vi "OFET.vi"() -> ()   [LabVIEW 2017]
uses:
  EnumEstados1.ctl
  <vilib>/Analysis/3filter.llb/Filter Passband Type.ctl
  <vilib>/Analysis/baseanly.llb/IIR Cascade Filter (DBL).vi
  <vilib>/Analysis/NI_AALBase.lvlib
  <vilib>/Utility/NIReport.llb/NI_report.lvclass
  <vilib>/addons/_office/NI_ReportGenerationToolkit.lvlib
  <vilib>/addons/_office/excel.llb/Excel Easy Table (str).vi
panel:
  in  "Tab Control":T1(tab)
  in  "Voltaje final:  2":dbl
  in  "Voltaje inicial:  2":dbl
  in  "Paso: 2":dbl
  in  "Voltaje final:":dbl
  in  "Voltaje inicial:":dbl
  in  "Paso:":dbl
  in  "Paso":dbl
  in  "Voltaje inicial:":dbl
  in  "Voltaje final:":dbl
  in  "Voltaje:":dbl
  in  "order":i32
  in  "Stop Button":bool
  in  "Save Button":bool
  in  "Guardar en:":path
  out "Voltage-Current Characterization:":cluster{dbl[], "Filtered X":dbl[]}(graph)
  in  "Ok":bool
  # "OFET"
  # "VGS"
  # "VDS"
  # "VGS"
  # "VDS"
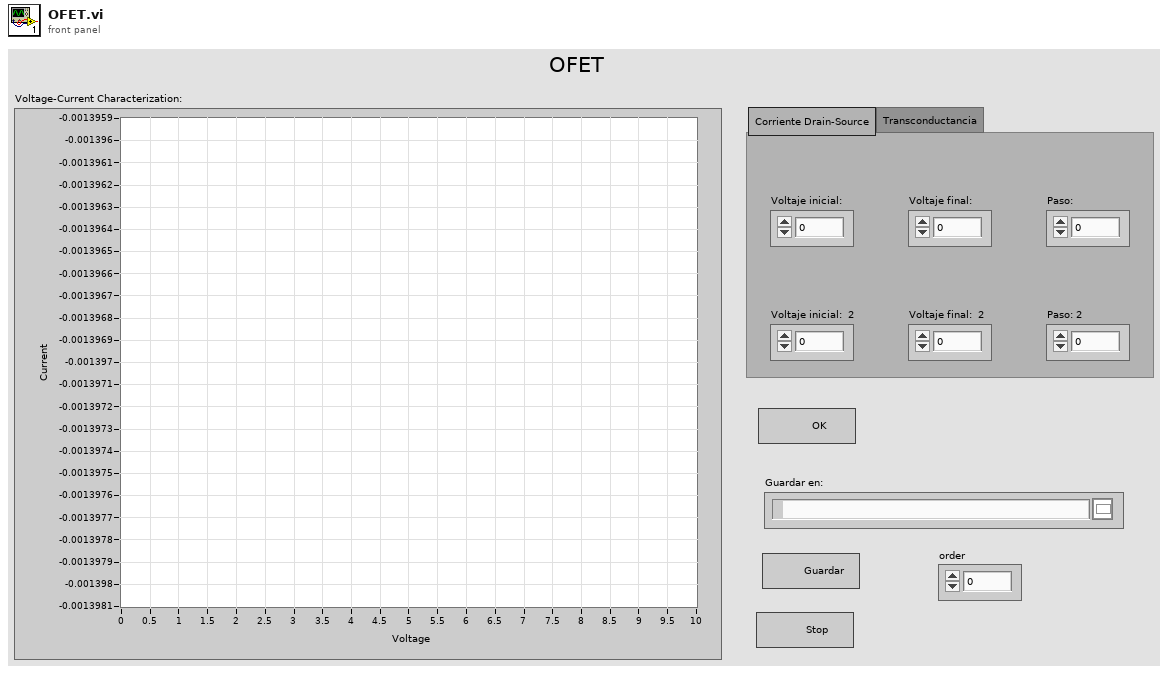
[diagram p1: front panel]
types:
  T1 = enum32{"Corriente Drain-Source", "Transconductancia"}
  T2 = typedef "EnumEstados1.ctl" = enum16{"Inicio", "LecturaDatos", "Cierre"}
  T3 = typedef "NI_AALBase.lvlib/Filter Passband Type.ctl" = enum32{"Lowpass", "Highpass", "Bandpass", "Bandstop"}
  T4 = enum16{"Standard Report", "HTML", "Word", "Excel"}
  T5 = enum16{"maximized", "minimized", "normal", "no change"}
  T6 = enum16{"open", "open or create", "create or replace", "create", "open (read-only)"}
  T7 = cluster{"task out":refnum<k21>, "error out":errorcluster}
  T8 = cluster{"filter structure":enum32{"IIR 2nd Order", "IIR 4th Order"}, "Reverse Coefficients":dbl[], "Forward Coefficients":dbl[]}
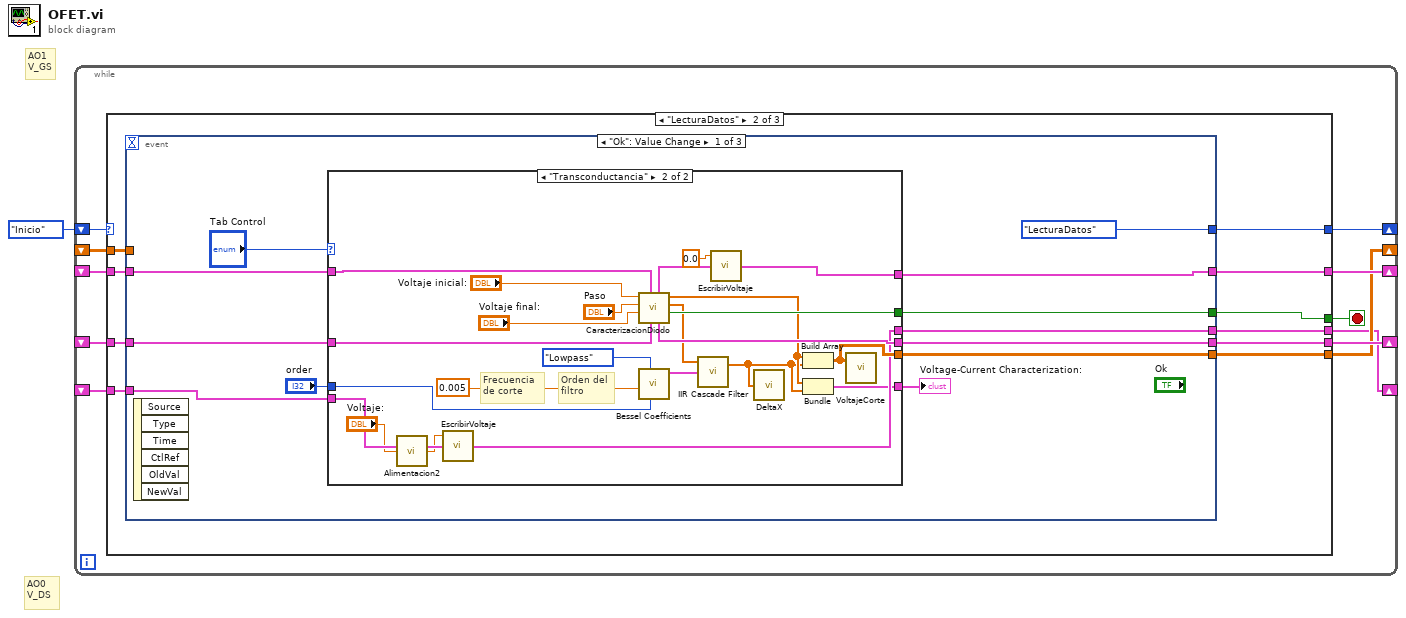
[diagram p0: block diagram]
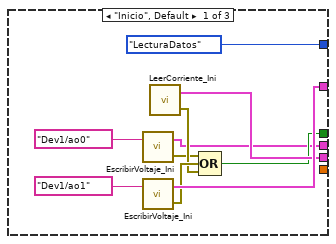
[diagram p2: hidden frame]
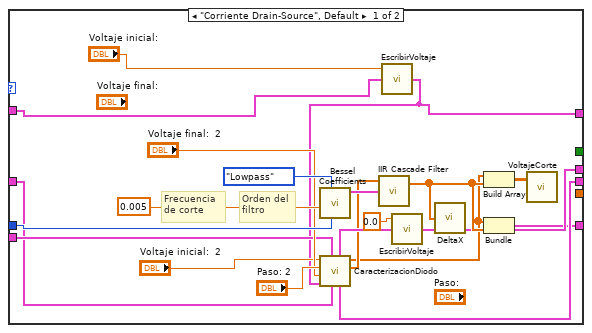
[diagram p3: hidden frame]
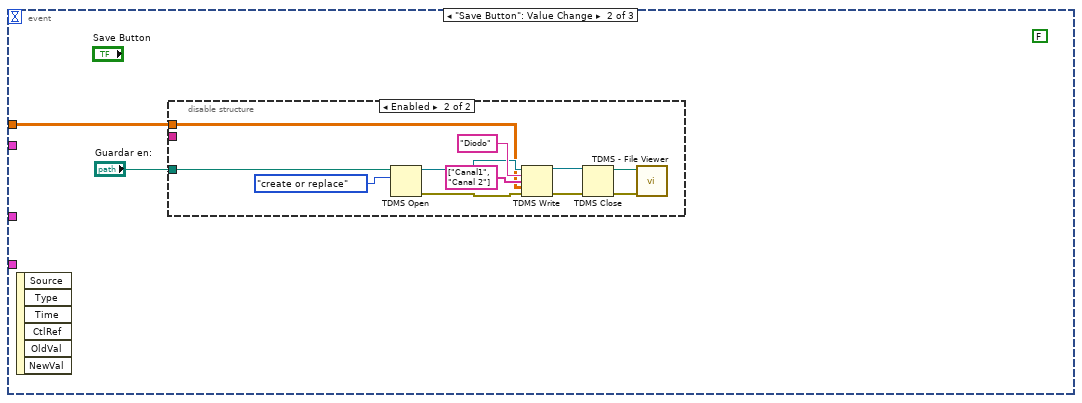
[diagram p4: hidden frame]
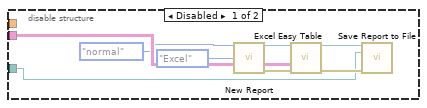
[diagram p5: hidden frame]
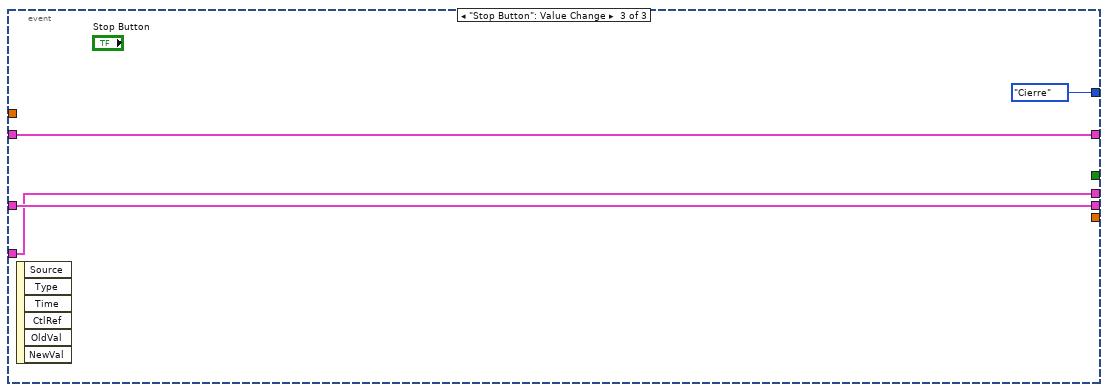
[diagram p6: hidden frame]
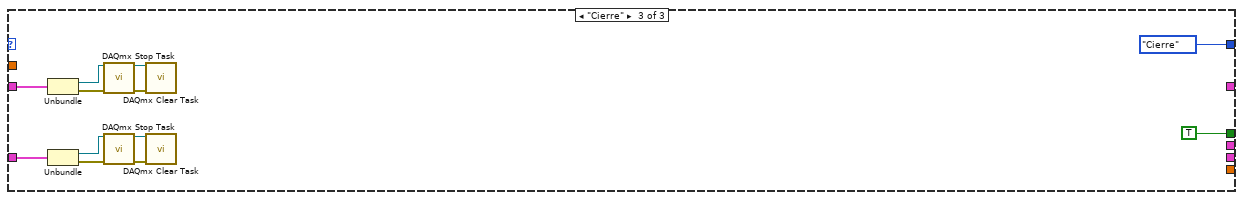
[diagram p7: hidden frame]
diagram:
  # "AO1\nV_GS"
  # "AO0\nV_DS"
  n1 = while {
    shift-right: [w7] -> _
    shift-left: EnumEstados1."Inicio" -> [w12]
    shift-right: [w11] -> _
    shift-left: _ -> [w10]
    shift-right: [w9] -> _
    shift-left: _ -> [w8]
    shift-right: [w6] -> _
    shift-left: _ -> [w5]
    shift-right: [w3] -> _
    shift-left: _ -> [w2]
    stop <- w4 stop-if-true
    n2 = case shown="\"LecturaDatos\"" w12 {
      tunnel: [w21 w31 _] -> w11
      tunnel: w10 -> [_ w32 w121]
      tunnel: [w20 w29 _] -> w9
      tunnel: w8 -> [_ w30 w120]
      tunnel: [EnumEstados1."LecturaDatos" w28 EnumEstados1."Cierre"] -> w7
      tunnel: [_ w27 _] -> w6
      tunnel: w5 -> [_ w26 _]
      tunnel: [w17 w25 TRUE] -> w4
      tunnel: [w16 w23 _] -> w3
      tunnel: w2 -> [_ w24 _]
      frame "Inicio", Default {
        n3 = call "EscribirVoltaje_Ini.vi"("physical channels"=tag "Dev1/ao0") -> ("error out"=w15:errorcluster, "cluster"=w16:T7)  [unwired: 1 in]
        n4 = call "EscribirVoltaje_Ini.vi"("physical channels"=tag "Dev1/ao1") -> ("error out"=w19:errorcluster, "cluster"=w21:T7)  [unwired: 1 in]
        n5 = call "LeerCorriente_Ini.vi"() -> ("error out"=w18:errorcluster, "output cluster"=w20:T7)  [unwired: 2 in]
        n6 = Compound Arithmetic op=OR(w15, w19, w18) -> (w17:bool)
      }
      frame "LecturaDatos" {
        n7 = event shown="[0] \"Ok\": Value Change" {
          selector: _ -> [_ _ _]
          dyn-events: _ -> [_ _ _]
          timeout: _ -> [_ _ _]
          tunnel: w32 -> [w43 _ w113]
          tunnel: [w36 _ w113] -> w31
          tunnel: w30 -> [w42 _ w112]
          tunnel: [w41 _ w112] -> w29
          tunnel: [EnumEstados1."LecturaDatos" _ EnumEstados1."Cierre"] -> w28
          tunnel: [w39 _ _] -> w27
          tunnel: w26 -> [_ w89 _]
          tunnel: [w40 _ _] -> w25
          tunnel: w24 -> [w38 _ w110]
          tunnel: [w37 _ w110] -> w23
          event "Ok": Value Change {
            n8 = event-data() -> ()  [unwired: 1 in, 6 out]
            n9 = case shown="\"Transconductancia\"" "Tab Control" {
              tunnel: w43 -> [w46 w86]
              tunnel: w42 -> [w55 w85]
              tunnel: [w54 w84] -> w41
              tunnel: [_ w83] -> w40
              tunnel: [_ w82] -> w39
              tunnel: w38 -> [w56 w78]
              tunnel: [w52 w77] -> w37
              tunnel: [w45 w75] -> w36
              tunnel: "order" -> [w60 w69]
              tunnel: [w48 w68] -> w33
              frame "Corriente Drain-Source", Default {
                # "Frecuencia \nde corte"
                # "Orden del\nfiltro"
                n10 = call <vilib>:"Bessel Coefficients.vi"("order"=w60, "filter type"=Filter_Passband_Type."Lowpass", "low cutoff freq: fl"=0.005 ("Numeric Control")) -> ("IIR Filter Cluster"=w65:T8)  [unwired: 7 in, 1 out]
                n11 = call "EscribirVoltaje.vi"("cluster"=w46, "data"="Voltaje inicial:") -> ("Cluster"=w45:T7)  [unwired: 1 in, 2 out]
                n12 = call "CaracterizacionDiodo.vi"("Corriente"=w55, "Voltaje"=w56, "Voltaje  2"=w45, "Voltaje final:"="Voltaje final:  2", "Paso"="Paso: 2", "Voltaje inicial:"="Voltaje inicial:  2") -> (2:"Corriente"=w50:dbl[], 3:"Voltaje"=w49:dbl[], 4:"Corriente"=w54:T7, 5:"Voltaje"=w53:T7)  [unwired: 1 in, 1 out]
                n13 = call-poly <vilib>:"IIR Cascade Filter.vi"("IIR Filter Cluster"=w65, "X"=w50) -> ("Filtered X"=w62:dbl[])  [unwired: 1 in, 1 out]
                n14 = call "EscribirVoltaje.vi"("cluster"=w53, "data"=0.0) -> ("Cluster"=w52:T7)  [unwired: 1 in, 2 out]
                n15 = call "DeltaX.vi"("Array in"=w62) -> ()  [unwired: 1 out]
                n16 = Build Array(w49, w62) -> (w63:dbl[][])
                n17 = Bundle("Voltaje"=w49, "Filtered X"=w62) -> (w48:cluster{"Voltaje":dbl[], "Filtered X":dbl[]})  [unwired: 1 in]
                n18 = call "VoltajeCorte.vi"("Array in"=w63) -> ()  [unwired: 1 in, 2 out]
              }
              frame "Transconductancia" {
                # "Frecuencia \nde corte"
                # "Orden del\nfiltro"
                n19 = call "Alimentacion2.vi"("VoltajeDeseado"="Voltaje:") -> ("Numeric Indicator"=w66:dbl)
                n20 = call "EscribirVoltaje.vi"("cluster"=w78, "data"=w66) -> ("Cluster"=w77:T7)  [unwired: 1 in, 2 out]
                n21 = call "CaracterizacionDiodo.vi"("Corriente"=w85, "Voltaje"=w86, "Voltaje final:"="Voltaje final:", "Paso"="Paso", "Voltaje inicial:"="Voltaje inicial:") -> ("Error?"=w83:bool, 2:"Corriente"=w73:dbl[], 3:"Voltaje"=w81:dbl[], 4:"Corriente"=w84:T7, 5:"Voltaje"=w76:T7)  [unwired: 2 in]
                n22 = call <vilib>:"Bessel Coefficients.vi"("order"=w69, "filter type"=Filter_Passband_Type."Lowpass", "low cutoff freq: fl"=0.005 ("Numeric Control")) -> ("IIR Filter Cluster"=w88:T8)  [unwired: 7 in, 1 out]
                n23 = call-poly <vilib>:"IIR Cascade Filter.vi"("IIR Filter Cluster"=w88, "X"=w73) -> ("Filtered X"=w80:dbl[])  [unwired: 1 in, 1 out]
                n24 = call "EscribirVoltaje.vi"("cluster"=w76, "data"=0.0) -> ("Cluster"=w75:T7)  [unwired: 1 in, 2 out]
                n25 = call "DeltaX.vi"("Array in"=w80) -> ()  [unwired: 1 out]
                n26 = Build Array(w81, w80) -> (w82:dbl[][])
                n27 = Bundle("Voltaje"=w81, "Filtered X"=w80) -> (w68:cluster{"Voltaje":dbl[], "Filtered X":dbl[]})  [unwired: 1 in]
                n28 = call "VoltajeCorte.vi"("Array in"=w82) -> ()  [unwired: 1 in, 2 out]
              }
            }
            "Voltage-Current Characterization:" <- w33
          }
          event "Save Button": Value Change {
            (unwired) FALSE
            n29 = event-data() -> ()  [unwired: 1 in, 6 out]
            n30 = disable-structure shown="Enabled" {
              disable-tunnel: _ -> [w96 _]
              disable-tunnel: "Guardar en:" -> [w91 w102]
              disable-tunnel: w89 -> [_ w99]
              frame Disabled {
                n31 = call <vilib>:"New Report.vi"("window state (normal)"=T5."normal", "report type"=T4."Excel") -> ("report out"=w98:refnum<class "NI_report.lvclass">, "error out"=w97:errorcluster)  [unwired: 12 in]
                n32 = call-poly <vilib>:"Excel Easy Table.vi"("report in"=w98, "text data"=w96, "error in (no error)"=w97) -> ("report out"=w95:refnum<class "NI_report.lvclass">, "error out"=w94:errorcluster)  [unwired: 8 in, 3 out]
                n33 = call-dynamic "Save Report to File.vi"("report in"=w95, "report file path"=w91, "error in (no error)"=w94) -> ()  [unwired: 11 in, 2 out]
              }
              frame Enabled {
                n34 = TDMS Open(10:T6."create or replace" ("operation (0:open)"), 11:w102) -> (0:w106:errorcluster, 3:w103:refnum<k34>)  [unwired: 5 in]
                n35 = TDMS Write(0:w103, 5:"Diodo" ("group name in (Untitled)"), 7:string[] ["Canal1", "Canal 2"] ("channel name(s) in (Untitled)"), 9:w99, 11:w106) -> (4:w104:refnum<k34>, 15:w105:errorcluster)  [unwired: 1 in, 2 out]
                n36 = TDMS Close(8:w105, 11:w104) -> (0:w101:errorcluster, 3:w100:path)
                n37 = call <vilib>:"TDMS - File Viewer.vi"("error in (no error)"=w101, "file path"=w100) -> ()  [unwired: 4 in, 2 out]
              }
            }
          }
          event "Stop Button": Value Change {
            n38 = event-data() -> ()  [unwired: 1 in, 6 out]
          }
        }
      }
      frame "Cierre" {
        n39 = Unbundle(w121) -> ("task out"=w119:refnum<k21>, "error out"=w118:errorcluster)
        n40 = Unbundle(w120) -> ("task out"=w117:refnum<k21>, "error out"=w116:errorcluster)
        n41 = call <vilib>:"DAQmx Stop Task.vi"("task/channels in"=w119, "error in"=w118) -> ("task out"=w125:refnum<k21>, "error out"=w124:errorcluster)  [unwired: 12 in]
        n42 = call <vilib>:"DAQmx Stop Task.vi"("task/channels in"=w117, "error in"=w116) -> ("task out"=w123:refnum<k21>, "error out"=w122:errorcluster)  [unwired: 12 in]
        n43 = call <vilib>:"DAQmx Clear Task.vi"("task in"=w125, "error in"=w124) -> ()  [unwired: 13 in, 1 out]
        n44 = call <vilib>:"DAQmx Clear Task.vi"("task in"=w123, "error in"=w122) -> ()  [unwired: 13 in, 1 out]
      }
    }
  }
